vi "Set Key.vi"(8 "error in (no error)":errorcluster, 9 "Define":bool=TRUE, 10 "Key":string, 11 "Stack in":T1[](array[typedef])) -> (0 "error out":errorcluster, 3 "Stack out":T1[](array[typedef]))   [LabVIEW 2020, in "TOML.lvlib"]
uses:
  TOML.lvlib
  Context.ctl
  Table Context.ctl
  Key-Value Pair.ctl
  Value.ctl
  Value Type.ctl
  Table Array Context.ctl
  <vilib>/ErrorRing/Error Ring.xnode
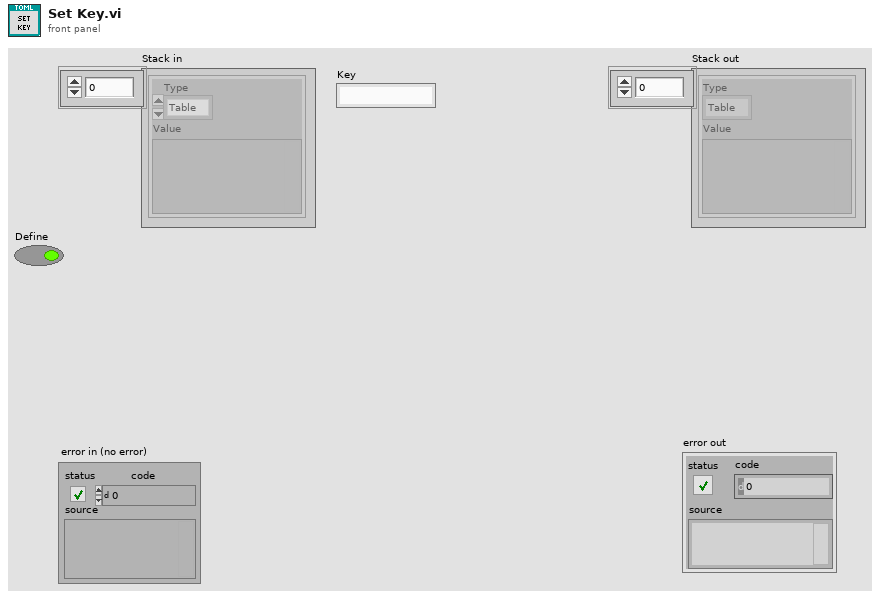
[diagram p1: front panel]
types:
  T1 = typedef "TOML.lvlib/Context.ctl" = cluster{"Type":enum16{"Table", "Array", "Inline Table", "Table Array"}, "Value":variant}
  T2 = typedef "TOML.lvlib/Table Context.ctl" = cluster{"Table":T3[], "Key":string, "Defined Keys":string[]}
  T3 = typedef "TOML.lvlib/Key-Value Pair.ctl" = cluster{"Key":string, "Value":T4}
  T4 = typedef "TOML.lvlib/Value.ctl" = cluster{"Type":T5, "Value":variant}
  T5 = typedef "TOML.lvlib/Value Type.ctl" = enum16{"Table", "Array", "String", "Integer", "Float", "Boolean", "Offset Date-Time", "Local Date-Time", "Local Date", "Local Time", "Path"}
  T6 = typedef "TOML.lvlib/Table Array Context.ctl" = cluster{"Table Array":cluster{"Table":T3[]}[], "Index":i32, "Key":string}
  T7 = enum16{"Table", "Array", "Inline Table", "Table Array"}
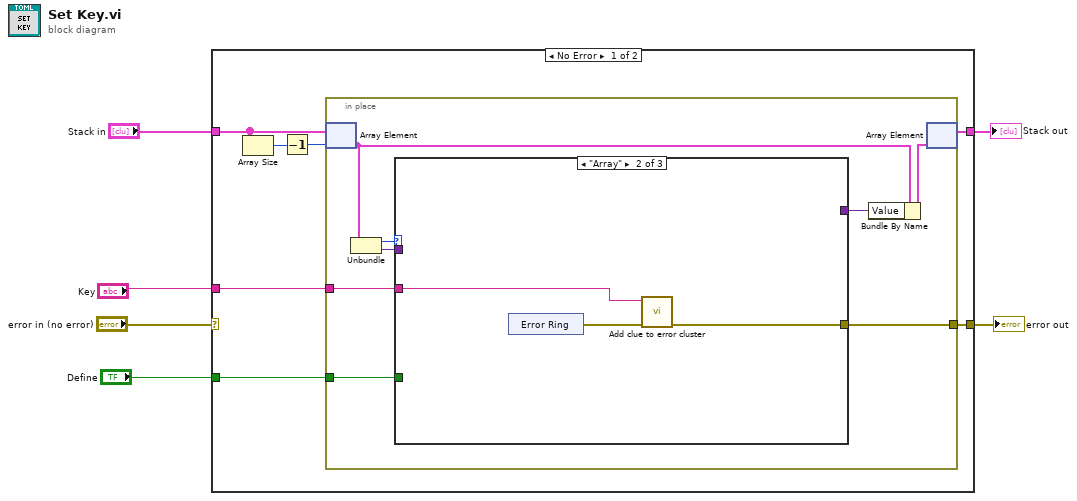
[diagram p0: block diagram]
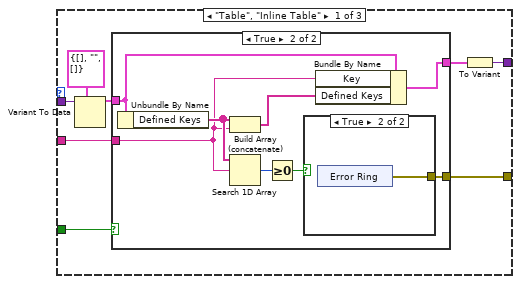
[diagram p2: hidden frame]
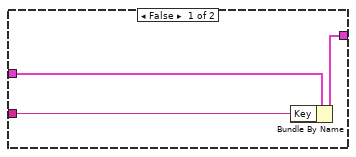
[diagram p3: hidden frame]
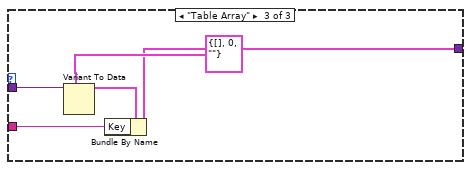
[diagram p5: hidden frame]
diagram:
  n1 = case shown="No Error" "error in (no error)" {
    selector: "error in (no error)" -> [_ w52]
    tunnel: "Stack in" -> [w11 w53]
    tunnel: [w10 w53] -> w5
    tunnel: "Key" -> [w9 _]
    tunnel: [w8 w52] -> w3
    tunnel: "Define" -> [w7 _]
    frame No Error {
      n2 = Array Size(array=w11) -> (size(s)=w13:i32)
      n3 = Decrement(x=w13) -> (x-1=w12:i32)
      n4 = in-place {
        in-place-border: w9 -> [w19]
        in-place-border: [w15] -> w8
        in-place-border: w7 -> [w14]
        n5 = in-place-array #1(w11, w12) -> (w18:T1)
        n6 = Unbundle(w18) -> ("Type"=w21:T7, "Value"=w20:variant)
        n7 = case shown="\"Array\"" w21 {
          tunnel: w20 -> [w23 _ w51]
          tunnel: w19 -> [w29 w43 w48]
          tunnel: [w27 _ w47] -> w17
          tunnel: [w22 w44 _] -> w15
          tunnel: w14 -> [w26 _ _]
          frame "Table", "Inline Table" {
            n8 = Variant To Data(type=T2 {"Table"=[], "Key"="", "Defined Keys"=[]} ("Table Context"), Variant=w23) -> (data=w24:T2)  [unwired: 1 in, 1 out]
            n9 = case shown="True" w26 {
              tunnel: w29 -> [w32 w36]
              tunnel: [w31 w34] -> w28
              tunnel: w24 -> [w30 w33]
              tunnel: [_ w37] -> w22
              frame False {
                n10 = Bundle By Name(cluster=w30, "Key"=w32) -> (w31:T2)
              }
              frame True {
                n11 = Unbundle By Name(w33) -> ("Defined Keys"=w40:string[])
                n12 = Build Array (concatenate)(w40, w36) -> (w35:string[])
                n13 = Search 1D Array(1D array=w40, element=w36) -> (index of element=w39:i32)  [unwired: 1 in]
                n14 = Greater Or Equal To 0?(x=w39) -> (x >= 0?=w38:bool)
                n15 = case shown="True" w38 {
                  tunnel: [_ w41] -> w37
                  frame False {
                  }
                  frame True {
                    n16 = xnode "Error Ring"() -> ("error out"=w41:errorcluster)
                  }
                }
                n17 = Bundle By Name(cluster=w33, "Key"=w36, "Defined Keys"=w35) -> (w34:T2)
              }
            }
            n18 = To Variant(anything=w28) -> (Variant=w27:variant)
          }
          frame "Array" {
            n19 = xnode "Error Ring"() -> ("error out"=w45:errorcluster)
            n20 = call "Add clue to error cluster.vi"("error in (no error)"=w45, "String"=w43) -> ("error out"=w44:errorcluster)  [unwired: 9 in]
          }
          frame "Table Array" {
            n21 = Variant To Data(type=T6 {"Table Array"=[], "Index"=0, "Key"=""} ("Table Array Context"), Variant=w51) -> (data=w49:T6)  [unwired: 1 in, 1 out]
            n22 = Bundle By Name(cluster=w49, "Key"=w48) -> (w47:T6)
          }
        }
        n23 = Bundle By Name(cluster=w18, "Value"=w17) -> (w16:T1)
        n24 = in-place-array #1(w16) -> (w10:T1[])  [unwired: 1 out]
      }
    }
    frame Error {
    }
  }
  "Stack out" <- w5
  "error out" <- w3
